vi "APU + Digital Pattern Sim.vi"() -> ()   [LabVIEW 2013]
uses:
  IP Source/Digital Pattern Generation/Load Input.ctl
  IP Source/Digital Pattern Generation/Input.ctl
  IP Source/Digital Pattern Generation/Settings.ctl
  IP Source/Version Token.ctl
  IP Source/APU/Shared Settings.ctl
  <vilib>/Platform/TimedLoop/XDataNode/timing_clust.ctl
  <vilib>/Platform/TimedLoop/XDataNode/nitl_modes.ctl
  <vilib>/Platform/TimedLoop/XDataNode/wakeup.ctl
  <vilib>/rvi/Emulation/niFpgaSctlEmulationGetInTimedLoop.vi
  <vilib>/rvi/Emulation/niFpgaEmulationReportErrorSimple.vi
  <vilib>/rvi/Emulation/niFpgaGetClockAttributes.vi
  <vilib>/rvi/Emulation/niFpgaCriticalErrorInLSC.vi
  <vilib>/rvi/DataTransferAndStorage/Container/Common/niFpgaContainerExecOnDevCompGetState.vi
  <vilib>/rvi/DataTransferAndStorage/Register/Emulation/niFpgaRegisterEmulationFpgaImpl.vi
  <instcachedir>/0/niFpgaRegisterEmulationFpgaImpl_DCF4BC0110594B98B44A971D60CEEC4D.lvgen/niFpgaRegisterEmulationFpgaImpl_DCF4BC0110594B98B44A971D60CEEC4D_006.vi
  <vilib>/rvi/DataTransferAndStorage/Container/Common/niFpgaContainerGetUniqueNameForEmu.vi
  <vilib>/rvi/DataTransferAndStorage/Container/Common/niFpgaContainerSetEmuInfo.vi
  <vilib>/rvi/eio/common/nirviEmuReportErrorAndStop.vi
  <vilib>/rvi/eio/common/nirviEmuTemplateMethod_errors.vi
  <vilib>/Platform/TimedLoop/XDataNode/XDataNode.xnode
  <vilib>/rvi/DataTransferAndStorage/Container/XNode/niFpgaContainer.xnode
  <vilib>/rvi/DataTransferAndStorage/Register/Emulation/niFpgaRegisterEmulationRefIn.vi
  <vilib>/rvi/LocalResourceManager/LocalResourceManager.xnode
  <vilib>/eio/EIONode/EIONode.xnode
  <vilib>/Platform/TimedLoop/XDataNode/XDNodeRunTimeDep.lvlib
  IP Source/APU/APU.lvlib
  IP Source/Digital Pattern Generation/Digital Pattern Generation.lvlib
  IP Source/Engine Simulation Toolkit.lvlib
panel:
  in  "shared settings.my apu":T1 {"start" format="%#.15g"}
  in  "eps.version":T2
  in  "Data":u16
  in  "settings.Pattern 1":T3
  in  "input.Pattern 1":T4
  in  "LoadInput.Pattern 1":T5
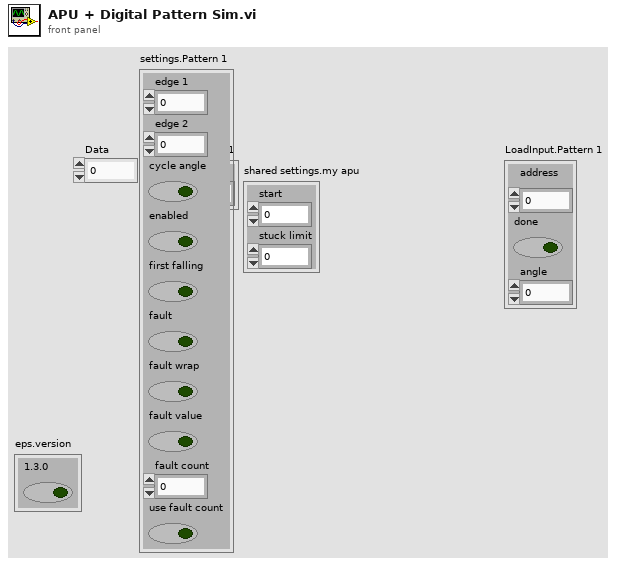
[diagram p1: front panel]
types:
  T1 = typedef "Engine Simulation Toolkit.lvlib/APU.lvlib/Shared Settings.ctl" = cluster{"start":fxp<+,17,17>, "stuck limit":fxp<+,18,18>}
  T2 = typedef "Engine Simulation Toolkit.lvlib/Version Token.ctl" = cluster{"1.3.0":bool}
  T3 = typedef "Engine Simulation Toolkit.lvlib/Digital Pattern Generation.lvlib/Settings.ctl" = cluster{"edge 1":u16, "edge 2":u16, "cycle angle":bool, "enabled":bool, "first falling":bool, "fault":bool, "fault wrap":bool, "fault value":bool, "fault count":fxp<+,4,4>, "use fault count":bool}
  T4 = typedef "Engine Simulation Toolkit.lvlib/Digital Pattern Generation.lvlib/Input.ctl" = cluster{"Offset":i16}
  T5 = typedef "Engine Simulation Toolkit.lvlib/Digital Pattern Generation.lvlib/Load Input.ctl" = cluster{"address":fxp<+,11,11>, "done":bool, "angle":u16}
  T6 = typedef "XDNodeRunTimeDep.lvlib/timing_clust.ctl" = cluster{"Expected End [f-1]":u64, "Actual End [f-1]":u64, "Finished Late? [f-1]":bool, "Expected End [i-1]":u64, "Actual End [i-1]":u64, "Finished Late? [i-1]":bool, "Expected Start [i]":u64, "Actual Start [i]":u64, "Expected Start [f]":u64, "Actual Start [f]":u64, "Source Name":string, "Structure Name":string, "Period":i64, "Deadline":i64, "Offset":i64, "Start":i64, "Priority":i32, "Timeout":i32, "Mode":T7, "Wakeup Reason":T8, "Error":errorcluster, "Source Type":string, "Secondary Source Type":string, "Global End Time":u64, "Global Start Time":u64, "Frame Duration":u64, "Iteration Duration":u64, "Assigned CPU":i32, "I/O Scan Engine Mode":u32}
  T7 = typedef "XDNodeRunTimeDep.lvlib/nitl_modes.ctl" = enum32{"No Change", "Process missed periods, maintain original phase", "Discard missed periods, maintain original phase", "Process missed periods, ignore original phase", "Discard missed periods, ignore original phase"}
  T8 = typedef "XDNodeRunTimeDep.lvlib/wakeup.ctl" = enum32{"Normal", "Aborted", "Asynchronous wakeup", "Timing source error", "Timed loop error", "Timeout"}
  T9 = typedef "Engine Simulation Toolkit.lvlib/Digital Pattern Generation.lvlib/Load Data.ctl" = cluster{"max address":fxp<+,11,11>, "memory":refnum<k21>}
  T10 = typedef "Engine Simulation Toolkit.lvlib/APU.lvlib/Register Bus.ctl" = cluster{"Speed":refnum<k21>, "Crank Angle":refnum<k21>, "Cycle Angle":refnum<k21>, "Crank Count":refnum<k21>, "Cycle Count":refnum<k21>, "1.25 MHz Counter":refnum<k21>, "Crank Rollover":refnum<k21>, "Cycle Rollover":refnum<k21>, "shared settings":T1}
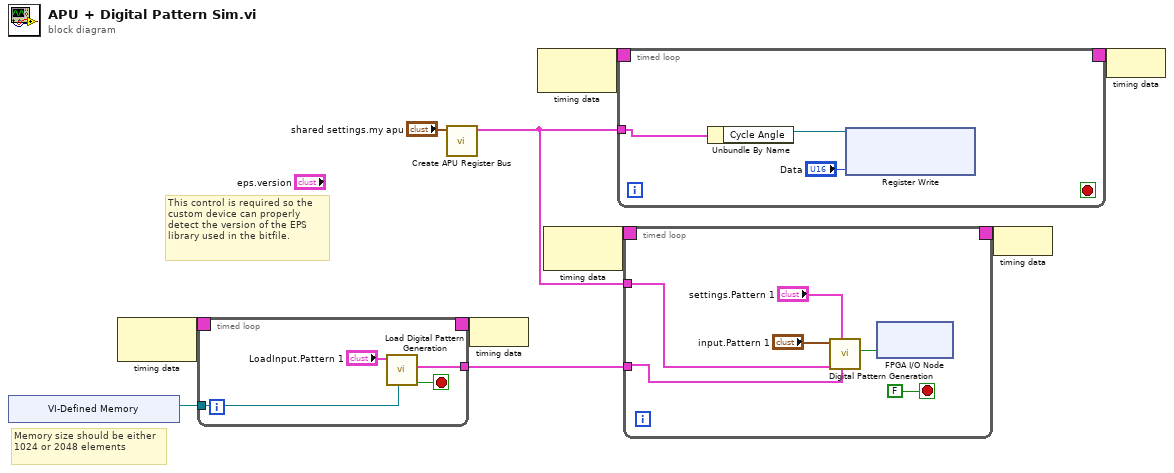
[diagram p0: block diagram]
diagram:
  # "This control is required so the custom device can properly detect the version of the EPS library used in the bitfile."
  # "Memory size should be either 1024 or 2048 elements"
  n1 = xnode "VI-Defined Memory"() -> ("Memory Out"=w6:refnum<k21>)
  n2 = node-c288() -> (w8:T6)  [unwired: 1 in]
  n3 = timed-loop {
    timing: w8 -> [_]
    timing-out: [_] -> w7
    tunnel: w6 -> [w13]
    tunnel: [w12] -> w2
    stop <- w14 stop-if-true
    n4 = call "Load Digital Pattern Generation.vi"("memory"=w13, "load input.<user name>"="LoadInput.Pattern 1") -> ("done"=w14:bool, "load data"=w12:T9)  [unwired: 8 in]
  }
  n5 = call "Create APU Register Bus.vi"("shared settings.<user name>"="shared settings.my apu") -> ("register bus"=w5:T10)  [unwired: 10 in]
  n6 = node-c288(w7) -> ()
  n7 = node-c288() -> (w10:T6)  [unwired: 1 in]
  n8 = node-c288() -> (w4:T6)  [unwired: 1 in]
  n9 = timed-loop {
    timing: w10 -> [_]
    timing-out: [_] -> w9
    tunnel: w5 -> [w19]
    stop <- _ stop-if-true
    n10 = Unbundle By Name(w19) -> ("Cycle Angle"=w18:refnum<k21>)
    n11 = xnode "Register Write"("Data"="Data", "Register In"=w18) -> ()  [unwired: 1 out]
  }
  n12 = timed-loop {
    tunnel: w5 -> [w23]
    timing: w4 -> [_]
    timing-out: [_] -> w3
    tunnel: w2 -> [w22]
    stop <- FALSE stop-if-true
    n13 = call "Digital Pattern Generation.vi"("load data"=w22, "settings.<user name>"="settings.Pattern 1", "register bus"=w23, "input.<user name>"="input.Pattern 1") -> ("digial output"=w25:bool)  [unwired: 7 in]
    n14 = xnode "FPGA I/O Node"("DO0"=w25) -> ()  [unwired: 1 in, 1 out]
  }
  n15 = node-c288(w3) -> ()
  n16 = node-c288(w9) -> ()
